vi "Close.vi"(8 "error in (no error)":errorcluster, 11 "VISA TCP Listener in":refnum<class "VISA TCP Listener.lvclass">) -> (0 "error out":errorcluster)   [LabVIEW 2013, in "Sockets.lvlib" / "VISA TCP Listener.lvclass"]
doc: "Closes a socket listener."
uses:
  VISA TCP Listener.lvclass
  VISA TCP Listener.lvclass/VISA TCP Listener.ctl
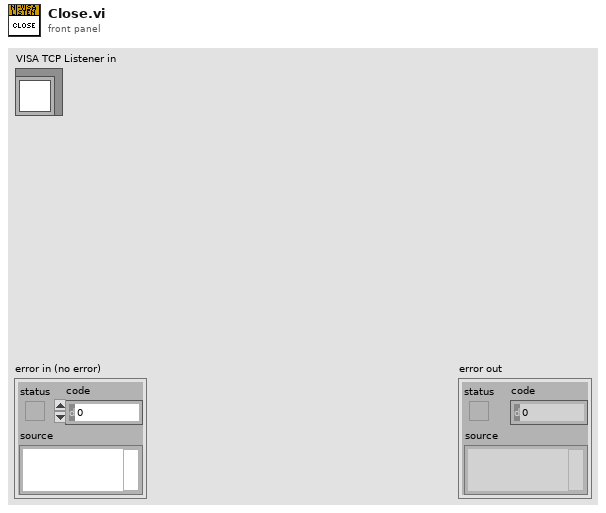
[diagram p1: front panel]
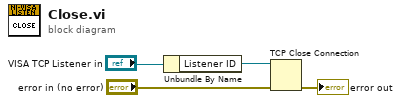
[diagram p0: block diagram]
diagram:
  n1 = Unbundle By Name("VISA TCP Listener in") -> ("Listener ID"=w3:refnum<k5>)
  n2 = TCP Close Connection(connection ID=w3, error in (no error)="error in (no error)") -> (error out=→"error out":errorcluster)  [unwired: 1 in, 1 out]
